vi "SubPanelVI1.vi"() -> ()   [LabVIEW 2016]
panel:
  in  "Stop":bool
  out "concatenated string":string
  in  "Concatenate":bool
  in  "String":string
  in  "Numeric":dbl
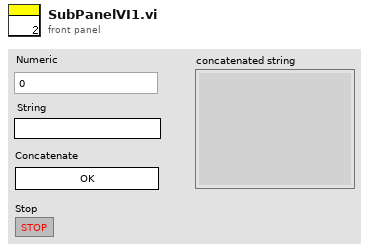
[diagram p1: front panel]
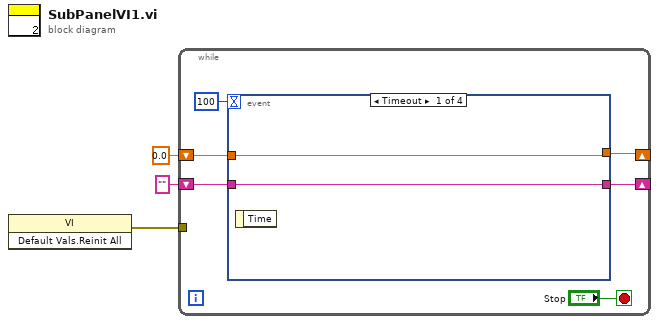
[diagram p0: block diagram]
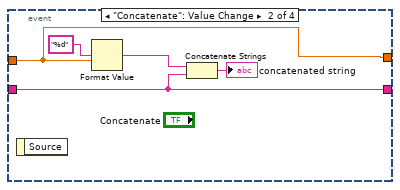
[diagram p2: hidden frame]
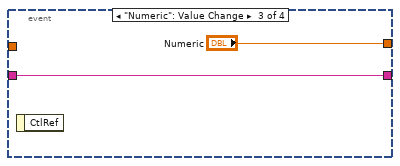
[diagram p3: hidden frame]
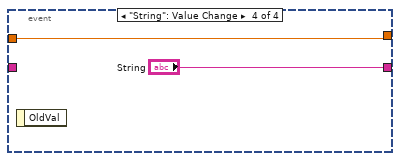
[diagram p4: hidden frame]
diagram:
  n1 = invoke class="VI" method="Default Vals.Reinit All"() -> (error out=w1:errorcluster)  [unwired: 3 in, 2 out]
  n2 = while {
    shift-right: [w8] -> _
    shift-left: "" ("String") -> [w6]
    shift-right: [w7] -> _
    shift-left: 0.0 ("Numeric") -> [w5]
    tunnel: w1 -> [_]
    stop <- "Stop" stop-if-true
    n3 = event shown="[0] Timeout" {
      selector: _ -> [_ _ _ _]
      dyn-events: _ -> [_ _ _ _]
      timeout: 100 -> [_ _ _ _]
      tunnel: [w11 w12 w17 "String"] -> w8
      tunnel: [w10 w13 "Numeric" w19] -> w7
      tunnel: w6 -> [w11 w12 w17 _]
      tunnel: w5 -> [w10 w13 _ w19]
      event Timeout {
        n4 = event-data() -> ()  [unwired: 1 in, 1 out]
      }
      event "Concatenate": Value Change {
        n5 = event-data() -> ()  [unwired: 1 in, 1 out]
        n6 = Format Value(format string="%d", value (0)=w13) -> (output string=w16:string)  [unwired: 1 in]
        n7 = Concatenate Strings(w16, w12) -> (→"concatenated string":string)
      }
      event "Numeric": Value Change {
        n8 = event-data() -> ()  [unwired: 1 in, 1 out]
      }
      event "String": Value Change {
        n9 = event-data() -> ()  [unwired: 1 in, 1 out]
      }
    }
  }
